vi "PH_Calorimeter_USB.panel.vi"(0 "object ref":refnum<vi>, 5 "error in (no error)":errorcluster) -> (19 "error out":errorcluster)   [LabVIEW 2014, in "PH_Calorimeter_USB.lvlib"]
doc: "By this VI a Calorimeter can be controlled. It gets the data from a USB device and calculates the energy from it.\n\n\n\n\nLicense Agreement for this software:\n\nCopyright (C)\nGesellschaft für Schwerionenforschung, GSI\nPlanckstr. 1\n64291 Darmstadt\nGermany\n\nContact: D.Beck@gsi.de \n\nThis program is free software; you can redistribute it and/or modify it under the terms of the GNU General Public License as published by the Free Software Foundation; either version 2 of the license, or (at your option) any later version.\n\nThis program is distributed in the hope that it will be useful, but WITHOUT ANYW ARRANTY; without even the implied warranty of MERCHANTABILITY or FITNESS FOR A PARTICULAR PURPOSE. See the GNU General License for more details (http://www.gnu.org).\n\nGesellschaft für Schwerionenforschung, GSI\nPlanckstr. 1, 64291 Darmstadt, Germany\nFor all questions and ideas contact: M.Richter@gsi.de, H.Brand@gsi.de or D.Beck@gsi.de.\nLast update: 18-DEC-2002"
uses:
  PH_Calorimeter_USB.lvlib
  PH_Calorimeter_USB.Calorimeter Settings.ctl
  PH_Calorimeter_USB.Trigger Settings.ctl
  PH_Calorimeter_USB.Time Base Settings.ctl
  PH_Calorimeter_USB.Calorimeter Calibration Settings.ctl
  CSCore/CSObj/CSObj.lvlib
  CSCore/CSSystem/CSSystemLib/CSSystemLib.lvlib
  PH_Common/PH_Common.lvlib
  PH_Class/PH_Class.lvlib
  PH_PSDBWriter/PH_PSDBWriter.lvlib
panel:
  out "PSDB Status":u32(colorbox)=6618880 caption="PSDB"
  out "Device":u32(colorbox)
  out "Calo Calibration":T1={"T 1/e [s]"=220.0, "Sensitivity  [Vs/J]"=0.0592} {"Sensitivity  [Vs/J]" format="%.4f"}
  out "Time Base":T2={"Samples per Channel"=28000, "Rate [Hz]"=100}
  out "Trigger":T3={"Channel"="", "Min Value [V]"=-10.0, "Max Value  [V]"=10.0, "Level [V]"=1.0, "Wait Time [s]"=60.0, "Length [Samples]"=10} {"Level [V]" format="%0.2f"; "Max Value  [V]" format="%0.2f"; "Min Value [V]" format="%0.2f"}
  out "Calorimeter":T4={"Channel"="Dev1/ai1", "Min Value [V]"=-1.0, "Max Value  [V]"=1.0} {"Max Value  [V]" format="%0.2f"; "Min Value [V]" format="%0.2f"}
  in  "Tab Control":enum32{"Result", "Raw Data"}(tab)
  out "Graph Result":cluster{dbl[], dbl[]}(graph)
  out "Graph Raw Data":dbl[][](graph)
  out "Energy":dbl caption="J" format="%.3f"
  in  "Start":bool
  in  "Exit":bool
  in  "Delete":bool
  # "PCS"
  # "3.40"
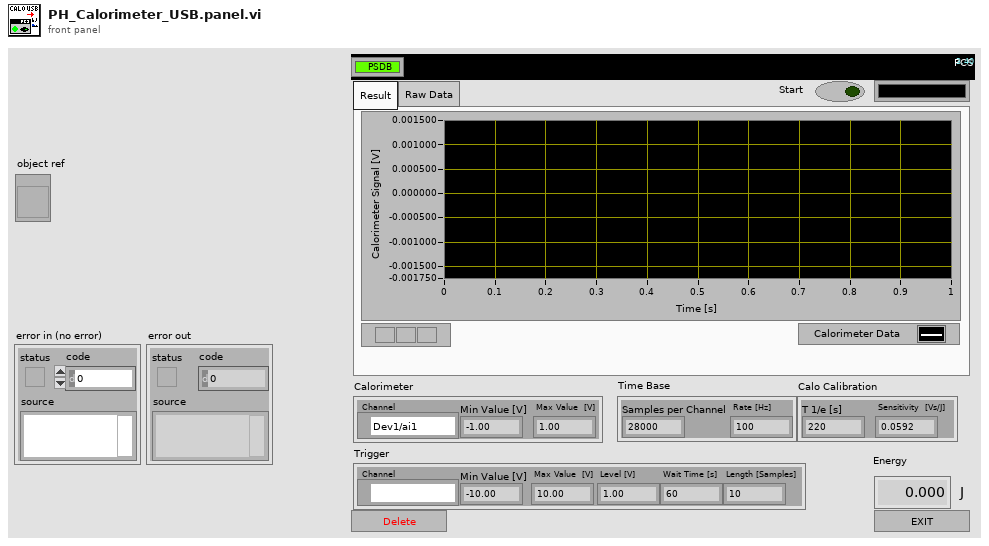
[diagram p1: front panel]
types:
  T1 = typedef "PH_Calorimeter_USB.lvlib/PH_Calorimeter_USB.Calorimeter Calibration Settings.ctl" = cluster{"T 1/e [s]":dbl, "Sensitivity  [Vs/J]":dbl}
  T2 = typedef "PH_Calorimeter_USB.lvlib/PH_Calorimeter_USB.Time Base Settings.ctl" = cluster{"Samples per Channel":i32, "Rate [Hz]":i32}
  T3 = typedef "PH_Calorimeter_USB.lvlib/PH_Calorimeter_USB.Trigger Settings.ctl" = cluster{"Channel":tag, "Min Value [V]":dbl, "Max Value  [V]":dbl, "Level [V]":dbl, "Wait Time [s]":dbl, "Length [Samples]":i32}
  T4 = typedef "PH_Calorimeter_USB.lvlib/PH_Calorimeter_USB.Calorimeter Settings.ctl" = cluster{"Channel":tag, "Min Value [V]":dbl, "Max Value  [V]":dbl}
  T5 = typedef "PH_Calorimeter_USB.lvlib/PH_Calorimeter_USB.i attribute.ctl" = cluster{"GUI Refs":cluster{"Delete":refnum<vi>, "Start":refnum<vi>, "Energy":refnum<vi>, "Calorimeter":refnum<vi>, "Trigger":refnum<vi>, "Calo Calibration":refnum<vi>, "Time Base":refnum<vi>, "Device":refnum<vi>, "Graph Raw Data":refnum<vi>, "Graph Result":refnum<vi>}, "DAQ Instance":string, "Data":dbl[][], "Controller Instance":string, "Energy [J]":dbl, "Calorimeter":T4, "Trigger":T3, "Time Base":T2, "Calo Calibration":T1, "Serial Number":string}
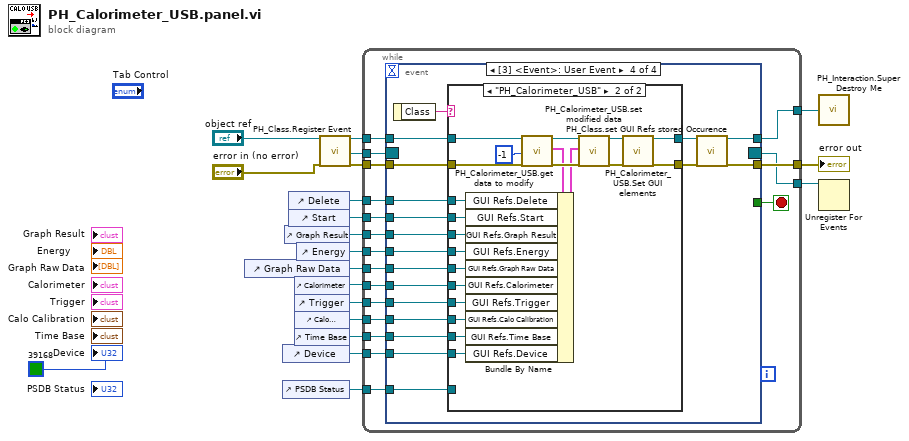
[diagram p0: block diagram]
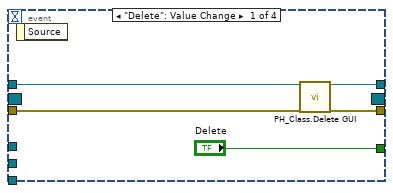
[diagram p2: hidden frame]
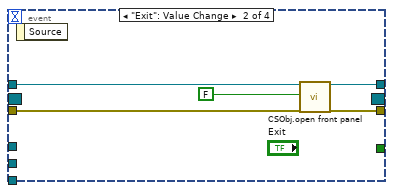
[diagram p3: hidden frame]
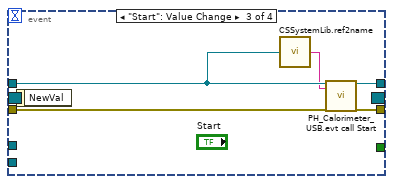
[diagram p4: hidden frame]
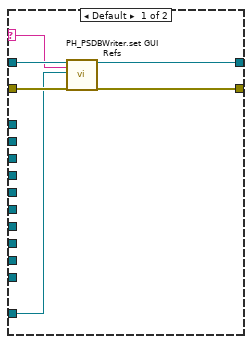
[diagram p5: hidden frame]
diagram:
  n1 = control-ref of="Graph Raw Data"() -> (w8:refnum<vi>)
  n2 = control-ref of="Device"() -> (w3:refnum<vi>)
  n3 = control-ref of="PSDB Status"() -> (w13:refnum<vi>)
  n4 = control-ref of="Graph Result"() -> (w10:refnum<vi>)
  n5 = control-ref of="Delete"() -> (w12:refnum<vi>)
  n6 = control-ref of="Start"() -> (w11:refnum<vi>)
  n7 = control-ref of="Calorimeter"() -> (w7:refnum<vi>)
  n8 = control-ref of="Trigger"() -> (w6:refnum<vi>)
  n9 = control-ref of="Calo Calibration"() -> (w5:refnum<vi>)
  n10 = control-ref of="Time Base"() -> (w4:refnum<vi>)
  n11 = control-ref of="Energy"() -> (w9:refnum<vi>)
  n12 = call "PH_Class.Register Event.vi"("i ref in"="object ref", "error in (no error)"="error in (no error)") -> ("i ref out"=w17:refnum<vi>, "Event Registration Refnum"=w15:refnum<event-registration>, "error out"=w16:errorcluster)  [unwired: 15 in]
  n13 = while {
    tunnel: w17 -> [w35]
    tunnel: [w34] -> w19
    tunnel: w16 -> [w37]
    tunnel: [w36] -> w18
    tunnel: w15 -> [w33]
    tunnel: [w32] -> w14
    tunnel: w13 -> [w31]
    tunnel: w12 -> [w30]
    tunnel: w11 -> [w29]
    tunnel: w10 -> [w28]
    tunnel: w9 -> [w27]
    tunnel: w8 -> [w26]
    tunnel: w7 -> [w25]
    tunnel: w6 -> [w24]
    tunnel: w5 -> [w23]
    tunnel: w4 -> [w22]
    tunnel: w3 -> [w21]
    stop <- w38 stop-if-true
    n14 = event shown="[3] <Event>: User Event" {
      selector: w33 -> [_ _ _ _]
      dyn-events: [_ _ _ _] -> w32
      timeout: _ -> [_ _ _ _]
      tunnel: ["Delete" _ _ _] -> w38
      tunnel: w35 -> [w42 w47 w53 w71]
      tunnel: w37 -> [w41 w46 w52 w70]
      tunnel: [w40 w45 w51 w66] -> w36
      tunnel: [w39 w44 w49 w67] -> w34
      tunnel: w31 -> [_ _ _ w64]
      tunnel: w30 -> [_ _ _ w63]
      tunnel: w29 -> [_ _ _ w62]
      tunnel: w28 -> [_ _ _ w61]
      tunnel: w27 -> [_ _ _ w60]
      tunnel: w26 -> [_ _ _ w59]
      tunnel: w25 -> [_ _ _ w58]
      tunnel: w24 -> [_ _ _ w57]
      tunnel: w23 -> [_ _ _ w56]
      tunnel: w22 -> [_ _ _ w55]
      tunnel: w21 -> [_ _ _ w54]
      event "Delete": Value Change {
        n15 = event-data() -> ()  [unwired: 1 in, 1 out]
        n16 = call "PH_Class.Delete GUI.vi"("VI in"=w42, "error in (no error)"=w41) -> ("VI out"=w39:refnum<vi>, "error out"=w40:errorcluster)  [unwired: 16 in]
      }
      event "Exit": Value Change {
        n17 = event-data() -> ()  [unwired: 1 in, 1 out]
        n18 = call "CSObj.open front panel.vi"("i ref in"=w47, "frontPanelOpen"=FALSE ("front panel open"), "error in (no error)"=w46) -> ("i ref out"=w44:refnum<vi>, "error out"=w45:errorcluster)  [unwired: 15 in]
      }
      event "Start": Value Change {
        n19 = event-data() -> ()  [unwired: 1 in, 1 out]
        n20 = call "CSSystemLib.ref2name.vi"("obj refnum"=w53) -> ("name"=w50:string)
        n21 = call "PH_Calorimeter_USB.evt call Start.vi"("i ref in"=w53, "Calorimeter Instance"=w50, "error in (no error)"=w52) -> ("i ref out"=w49:refnum<vi>, "error out"=w51:errorcluster)  [unwired: 15 in]
      }
      event User Event {
        n22 = event-data() -> ("Class"=w65:string)  [unwired: 1 in]
        n23 = case shown="\"PH_Calorimeter_USB\"" w65 {
          selector: w65 -> [w73 _]
          tunnel: w71 -> [w77 w93]
          tunnel: w70 -> [w76 w92]
          tunnel: [w74 w79] -> w69
          tunnel: [w75 w78] -> w68
          tunnel: w64 -> [w72 _]
          tunnel: w63 -> [_ w91]
          tunnel: w62 -> [_ w90]
          tunnel: w61 -> [_ w89]
          tunnel: w60 -> [_ w88]
          tunnel: w59 -> [_ w87]
          tunnel: w58 -> [_ w86]
          tunnel: w57 -> [_ w85]
          tunnel: w56 -> [_ w84]
          tunnel: w55 -> [_ w83]
          tunnel: w54 -> [_ w82]
          frame Default {
            n24 = call "PH_PSDBWriter.set GUI Refs.vi"("i ref in"=w77, "Class"=w73, "Ref PSDB Status"=w72, "error in"=w76) -> ("i ref out"=w75:refnum<vi>, "error out"=w74:errorcluster)  [unwired: 14 in]
          }
          frame "PH_Calorimeter_USB" {
            n25 = call "PH_Calorimeter_USB.get data to modify.vi"("i ref in"=w93, "ms timeout (10000)"=-1, "error in (no error)"=w92) -> ("i ref out"=w98:refnum<vi>, "i attribute"=w94:T5, "error out"=w97:errorcluster)  [unwired: 13 in, 1 out]
            n26 = Bundle By Name(cluster=w94, "GUI Refs.Delete"=w91, "GUI Refs.Start"=w90, "GUI Refs.Graph Result"=w89, "GUI Refs.Energy"=w88, "GUI Refs.Graph Raw Data"=w87, "GUI Refs.Calorimeter"=w86, "GUI Refs.Trigger"=w85, "GUI Refs.Calo Calibration"=w84, "GUI Refs.Time Base"=w83, "GUI Refs.Device"=w82) -> (w95:T5)
            n27 = call "PH_Calorimeter_USB.set modified data.vi"("i ref in"=w98, "i attribute"=w95, "error in (no error)"=w97) -> ("i ref out"=w80:refnum<vi>, "error out"=w81:errorcluster)  [unwired: 15 in]
            n28 = call "PH_Calorimeter_USB.Set GUI elements.vi"("i ref in"=w80, "error in (no error)"=w81) -> ("i ref out"=w78:refnum<vi>, "error out"=w79:errorcluster)  [unwired: 16 in]
          }
        }
        n29 = call "PH_Class.set GUI Refs stored Occurence.vi"("i ref in"=w68, "error in (no error)"=w69) -> ("i ref out"=w67:refnum<vi>, "error out"=w66:errorcluster)  [unwired: 16 in]
      }
    }
  }
  "error out" <- w18
  n30 = call "PH_Interaction.Super Destroy Me.vi"("i ref out"=w19) -> ()
  n31 = Unregister For Events(event registration refnum=w14) -> ()  [unwired: 1 in, 1 out]
  "Device" <- u32 39168 ("Device")
